vi "SP - get cluster details.vi"(8 "error in (no error)":errorcluster, 11 "JSON string":string) -> (0 "error out":errorcluster, 3 "value":string)   [LabVIEW 2020, in "ui-testing.lvlib"]
doc: "copyright: Thomas Zilliox©"
uses:
  ui-testing.lvlib
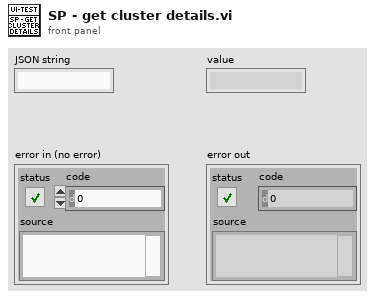
[diagram p1: front panel]
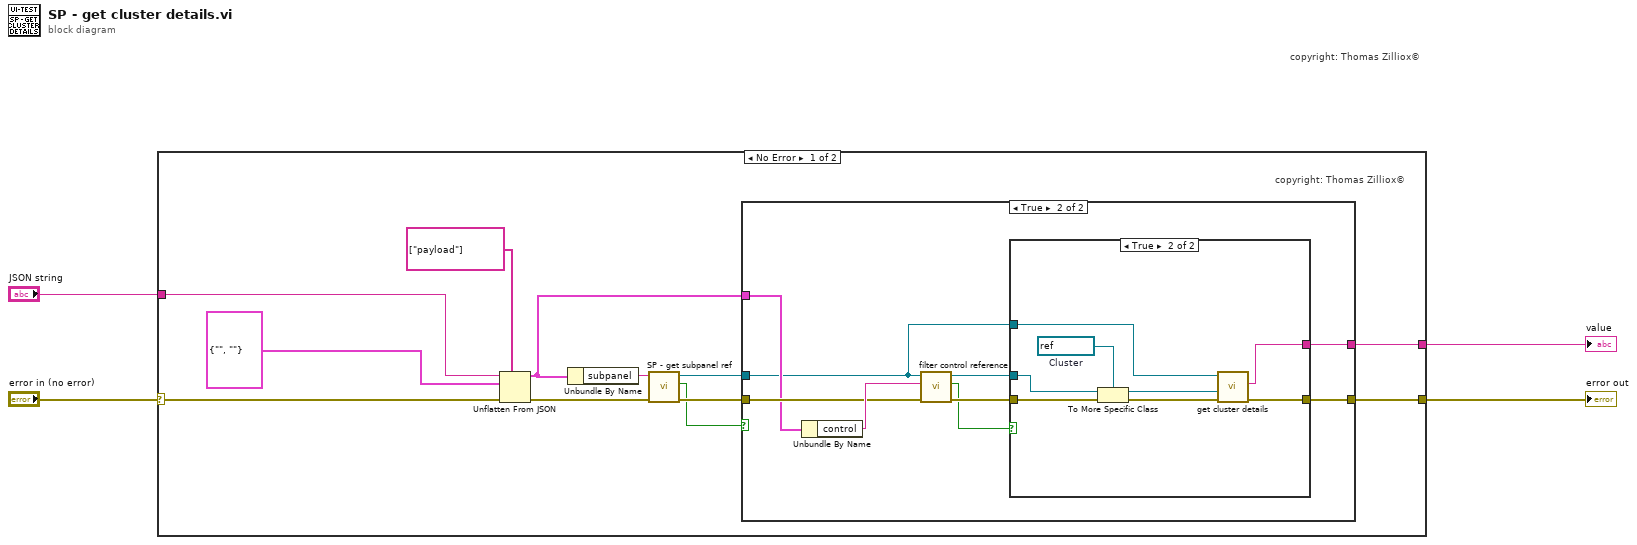
[diagram p0: block diagram]
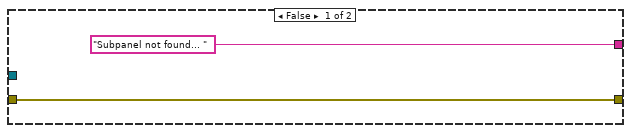
[diagram p2: hidden frame]
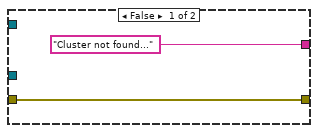
[diagram p3: hidden frame]
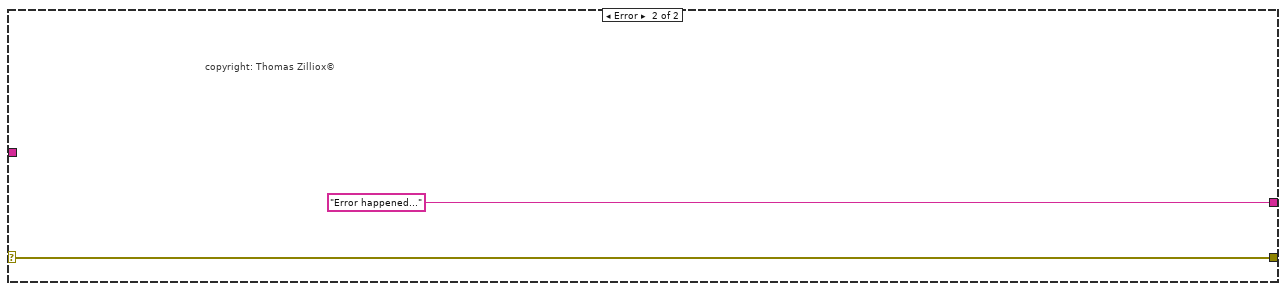
[diagram p4: hidden frame]
diagram:
  # "copyright: Thomas Zilliox©"
  n1 = case shown="No Error" "error in (no error)" {
    selector: "error in (no error)" -> [w14 w39]
    tunnel: "JSON string" -> [w15 _]
    tunnel: [w11 w39] -> w3
    tunnel: [w12 "Error happened..."] -> w2
    frame No Error {
      # "copyright: Thomas Zilliox©"
      n2 = Unflatten From JSON(path=string[] ["payload"], JSON string=w15, type and defaults=cluster{"control":string, "subpanel":string} {"control"="", "subpanel"=""}, error in (no error)=w14) -> (value=w7:cluster{"control":string, "subpanel":string}, error out=w10:errorcluster)  [unwired: 3 in]
      n3 = Unbundle By Name(w7) -> ("subpanel"=w6:string)
      n4 = call "SP - get subpanel ref.vi"("error in (no error)"=w10, "subpanel"=w6) -> ("error out"=w9:errorcluster, "subpanel found ?"=w5:bool, "subpanel VI ref"=w8:refnum<vi>)  [unwired: 6 in, 1 out]
      n5 = case shown="True" w5 {
        tunnel: ["Subpanel not found... " ("result string") w23] -> w12
        tunnel: [w17 w22] -> w11
        tunnel: w9 -> [w17 w21]
        tunnel: w8 -> [_ w19]
        tunnel: w7 -> [_ w20]
        frame False {
        }
        frame True {
          n6 = Unbundle By Name(w20) -> ("control"=w27:string)
          n7 = call "filter control reference.vi"("error in (no error)"=w21, "Control label"=w27, "VI (Caller)"=w19) -> ("error out"=w25:errorcluster, "Control found"=w24:bool, "Control ref"=w26:refnum<vi>)  [unwired: 6 in]
          n8 = case shown="True" w24 {
            tunnel: w26 -> [_ w36]
            tunnel: w25 -> [w29 w37]
            tunnel: [w29 w30] -> w22
            tunnel: ["Cluster not found..." w32] -> w23
            tunnel: w19 -> [_ w33]
            frame False {
            }
            frame True {
              w35 = refnum<vi> refnum  # Cluster
              n9 = To More Specific Class(target class=w35, reference=w36, error in=w37) -> (specific class reference=w34:refnum<vi>, error out=w31:errorcluster)
              n10 = call "get cluster details.vi"("error in"=w31, "Cluster-target"=w34, "VI Refnum"=w33) -> ("error out"=w30:errorcluster, "Control details"=w32:string)  [unwired: 7 in]
            }
          }
        }
      }
    }
    frame Error {
      # "copyright: Thomas Zilliox©"
    }
  }
  "error out" <- w3
  "value" <- w2
